vi "DeInit.vi"(8 "error in (no error)":errorcluster, 11 "HamaCam in":refnum<class "HamaCam.lvclass">) -> (0 "error out":errorcluster, 3 "HamaCam out":refnum<class "HamaCam.lvclass">)   [LabVIEW 2023, in "HamaCam.lvlib" / "HamaCam.lvclass"]
uses:
  HamaCam.lvclass
  HamaCam.lvclass/HamaCam.ctl
  <vilib>/ActorFramework/Actor/Actor.lvclass
  Applications/National Instruments/LabVIEW 2023 64-bit/vi.lib/ActorFramework/Actor/Actor.lvclass
  Users/alexandrosspiliotis/Documents/LV_DAQ_Project/ConcreteClasses/ConcreteInstrumentClasses/CameraClasses/Hama_LV/HamaCam/HamaCam/HamaCam.lvclass
  Users/alexandrosspiliotis/Documents/LV_DAQ_Project/Interfaces/AbstractInstrumentClasses/Cameras_LV/CameraInterface/CameraInterface.lvclass
  Users/alexandrosspiliotis/Documents/LV_DAQ_Project/Interfaces/InitDeinitInterface/InitDeinit/InitDeinit.lvclass
  Interfaces/InitDeinitInterface/InitDeinitComm Messages/InitDone Msg/InitDone Msg.lvclass
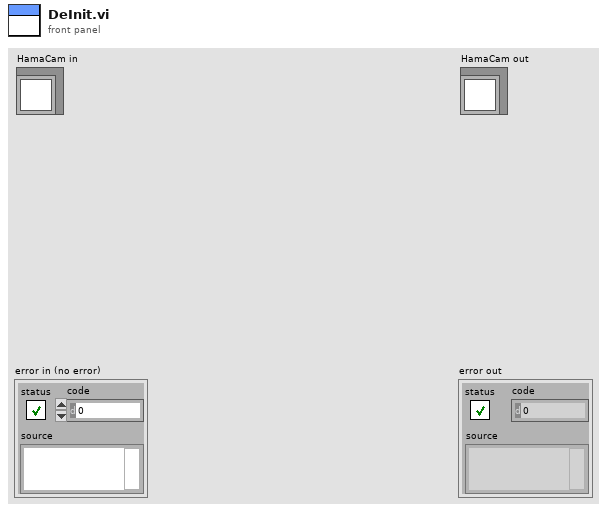
[diagram p1: front panel]
types:
  T1 = typedef "SpectroscopyUI.lvlib/InstrumentData.ctl" = cluster{"Instr Error":errorcluster, "Address":cluster{"address type":enum16{"VISA", "Index"}, "Address":string, "instrument type":T2}, "CurrentState":cluster{"Initialized":bool, "Connected":bool, "Running":bool, "Error":bool}, "Enqueuer":refnum<class "Message Enqueuer.lvclass">}
  T2 = typedef "instrumentType.ctl" = enum16{"Spectrometer", "Camera", "Stepper"}
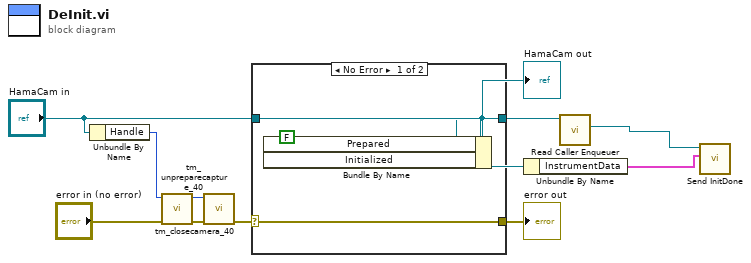
[diagram p0: block diagram]
diagram:
  n1 = Unbundle By Name("HamaCam in") -> ("Handle"=w8:u32)
  n2 = call "tm_unpreparecapture_40.vi"("error in (no error)"="error in (no error)", "Handle in"=w8) -> ("error out"=w10:errorcluster, "Handle out"=w9:u32)  [unwired: 8 in]
  n3 = call "tm_closecamera_40.vi"("error in (no error)"=w10, "Handle in"=w9) -> ("error out"=w6:errorcluster)  [unwired: 9 in]
  n4 = case shown="No Error" w6 {
    selector: w6 -> [w11 w15]
    tunnel: "HamaCam in" -> [w14 w16]
    tunnel: [w13 w16] -> w3
    tunnel: [w11 w15] -> w4
    frame No Error {
      w12 = FALSE ("CurrentState.Initialized")
      n5 = Bundle By Name(cluster=w14, "Prepared"=w12, "Initialized"=w12) -> (w13:refnum<class "HamaCam.lvclass">)
    }
    frame Error {
    }
  }
  "HamaCam out" <- w3
  "error out" <- w4
  n6 = Unbundle By Name(w3) -> ("InstrumentData"=w1:T1)
  n7 = call <vilib>:"Read Caller Enqueuer.vi"("Actor"=w3) -> ("Caller Enqueuer"=w2:refnum<class "Message Enqueuer.lvclass">)  [unwired: 10 in]
  n8 = call "Send InitDone.vi"("InstrumentData"=w1, "Message Enqueuer"=w2) -> ()  [unwired: 8 in, 2 out]
